vi "Search File.vi"(0 "Path":path, 1 "File Name":string) -> (14 "New Path":path, 15 "File Found?":bool)   [LabVIEW 2019]
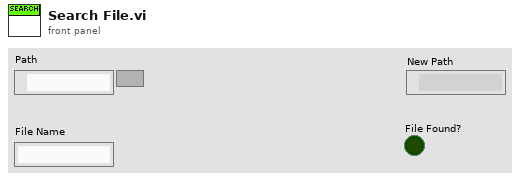
[diagram p1: front panel]
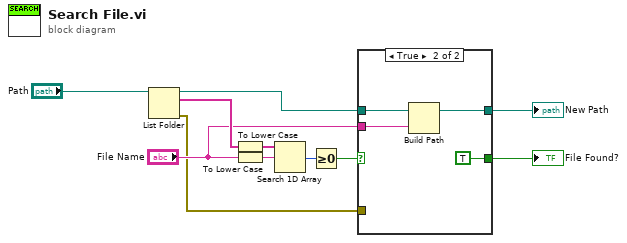
[diagram p0: block diagram]
diagram:
  n1 = List Folder(path="Path") -> (path out=w6:path, filenames=w8:string[], error out=w1:errorcluster)  [unwired: 3 in, 1 out]
  n2 = To Lower Case(string=w8) -> (all lower case string=w9:string[])
  n3 = To Lower Case(string="File Name") -> (all lower case string=w10:string)
  n4 = Search 1D Array(1D array=w9, element=w10) -> (index of element=w11:i32)  [unwired: 1 in]
  n5 = Greater Or Equal To 0?(x=w11) -> (x >= 0?=w4:bool)
  n6 = case shown="True" w4 {
    selector: w4 -> [w12 _]
    tunnel: w6 -> [w13 w17]
    tunnel: "File Name" -> [_ w16]
    tunnel: [w13 w15] -> w3
    tunnel: [w12 TRUE ("File Found?")] -> w2
    tunnel: w1 -> [_ _]
    frame False {
    }
    frame True {
      n7 = Build Path(base path=w17, name or relative path=w16) -> (appended path=w15:path)
    }
  }
  "File Found?" <- w2
  "New Path" <- w3
